vi "network_apply.vi"(8 "error":errorcluster, 11 "connection ID":refnum<k5>) -> (0 "error out":errorcluster, 3 "connection ID out":refnum<k5>)   [LabVIEW 2016, in "sen_api.lvlib"]
doc: "Applies the temporary IP configuration and loads it."
uses:
  sen_api.lvlib
panel:
  out "jsonRespIn":string
  out "JSON-response":string="{\"jsonrpc\":\"2.0\",\"method\":\"\",\"params\":[5,1.245,true,\"name\"],\"id\":\"1\"}"
  out "JSON request":string
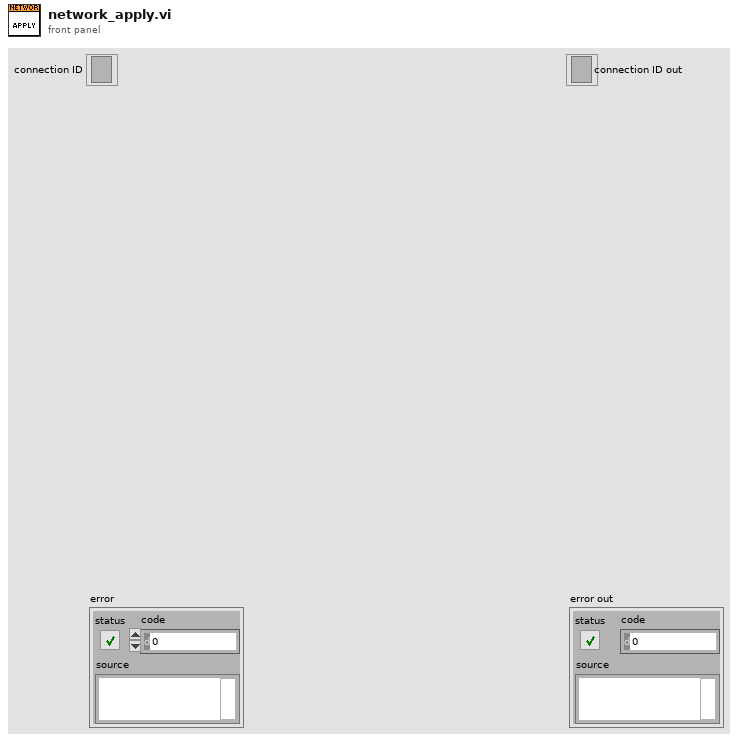
[diagram p1: front panel]
types:
  T1 = cluster{"jsonrpc":string, "method":string, "params":string[], "id":string, "api":i32, "pid":string}
  T2 = enum16{"Standard", "Buffered", "CRLF", "Immediate"}
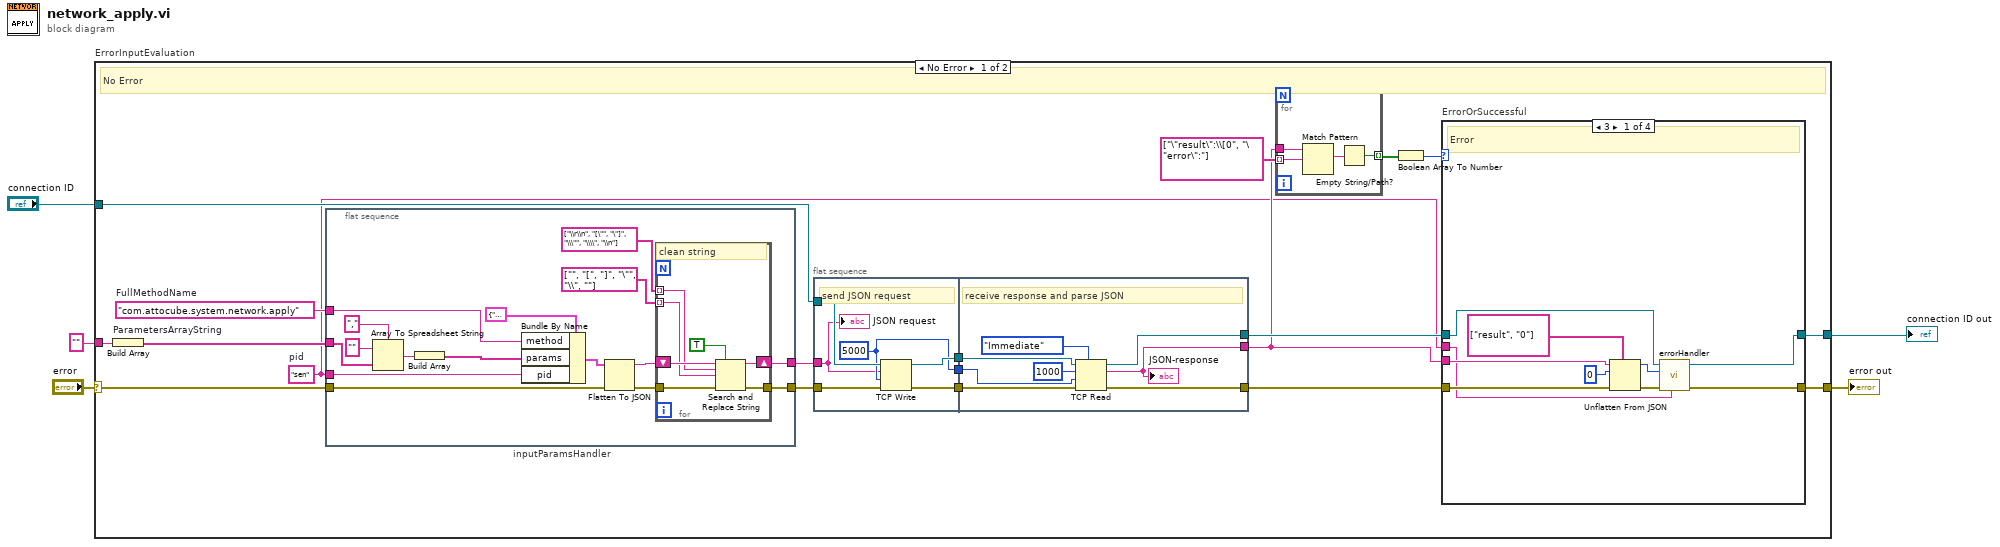
[diagram p0: block diagram]
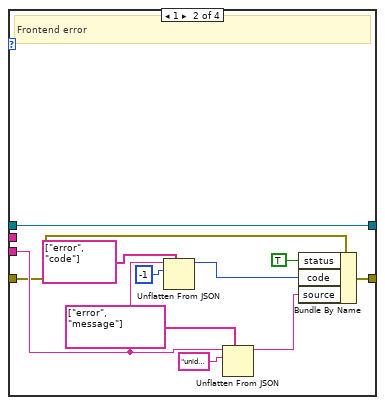
[diagram p2: hidden frame]
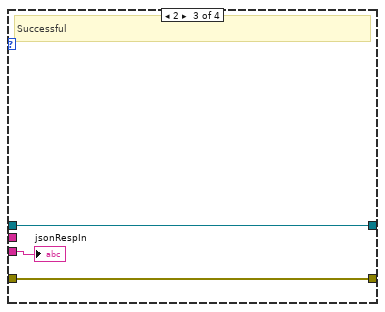
[diagram p3: hidden frame]
diagram:
  n1 = case "ErrorInputEvaluation" shown="No Error" "error" {
    selector: "error" -> [w11 w92]
    tunnel: "connection ID" -> [w21 w93]
    tunnel: [w13 w92] -> w4
    tunnel: [w14 w93] -> w3
    tunnel: "" -> [w6 _]
    frame No Error {
      w7 = "sen"  # pid
      w12 = "com.attocube.system.network.apply"  # FullMethodName
      # "No Error"
      n2 = Build Array "ParametersArrayString"(w6) -> (w10:string[])
      n3 = flat-sequence "inputParamsHandler" {
        tunnel: [w28] -> w9
        tunnel: w10 -> [w35]
        tunnel: w11 -> [w33]
        tunnel: [w30] -> w8
        tunnel: w12 -> [w36]
        tunnel: w7 -> [w25]
        frame #0 {
          n4 = Array To Spreadsheet String(delimiter (Tab)=",", array=w35, 3:"" ("format string")) -> (spreadsheet string=w38:string)
          n5 = Build Array "Build Array"(w38) -> (w34:string[])
          n6 = Bundle By Name(cluster=T1 {"jsonrpc"="2.0", "method"="com.attocube.amc.res.setRESReadOutFreq", "params"=[], "id"="1", "api"=2, "pid"=""}, "method"=w36, "params"=w34, "pid"=w25) -> (w37:T1)
          n7 = Flatten To JSON(anything=w37, error in (no error)=w33) -> (JSON string=w29:string, 11:w31:errorcluster)  [unwired: 1 in]
          n8 = for {
            tunnel: string[] ["\\r\\n", "[\"", "\"]", "\\\"", "\\\\", "\\n"] ("search string") -> [w44] mode=indexing
            tunnel: string[] ["", "[", "]", "\"", "\\", ""] ("replace string (\"\")") -> [w43] mode=indexing
            shift-right: [w46] -> w28
            shift-left: w29 -> [w45]
            tunnel: w31 -> [w42]
            tunnel: [w41] -> w30
            # "clean string"
            n9 = Search and Replace String(replace all?=TRUE ("replace all? (F)"), input string=w45, search string=w44, replace string=w43, error in=w42) -> (result string=w46:string, error out=w41:errorcluster)  [unwired: 3 in, 2 out]
          }
        }
      }
      n10 = flat-sequence {
        tunnel: w21 -> [w83]
        tunnel: [w81] -> w24
        tunnel: [w82] -> w23
        tunnel: w8 -> [w78]
        tunnel: [w80] -> w22
        tunnel: w9 -> [w79]
        tunnel: [w87] -> w17
        tunnel: w24 -> [w89]
        tunnel: w23 -> [w88]
        tunnel: [w85] -> w16
        tunnel: w22 -> [w86]
        tunnel: [w84] -> w15
        frame #0 {
          w80 = 5000 ("timeout ms (25000)")
          # "send JSON request"
          n11 = TCP Write(connection ID=w83, data in=w79, error in (no error)=w78, 9:w80) -> (connection ID out=w81:refnum<k5>, error out=w82:errorcluster)  [unwired: 1 out]
          "JSON request" <- w79
        }
        frame #1 {
          # "receive response and parse JSON"
          n12 = TCP Read(connection ID=w89, bytes to read=1000, error in (no error)=w88, 7:T2."Immediate" ("mode (standard)"), 9:w86) -> (connection ID out=w87:refnum<k5>, data out=w84:string, error out=w85:errorcluster)
          "JSON-response" <- w84
        }
      }
      n13 = for {
        tunnel: string[] ["\"result\":\\[0", "\"error\":"] ("path") -> [w50] mode=indexing
        tunnel: [w48] -> w19 mode=indexing
        tunnel: w15 -> [w51]
        n14 = Match Pattern(string=w51, regular expression=w50) -> (match substring=w49:string)  [unwired: 1 in, 3 out]
        n15 = Empty String/Path?(string/path=w49) -> (empty?=w48:bool)
      }
      n16 = Boolean Array To Number(Boolean array=w19) -> (number=w18:u32)
      n17 = case "ErrorOrSuccessful" shown="3" w18 {
        tunnel: w15 -> [w55 w64 w73 _]
        tunnel: w17 -> [w59 w62 w75 w77]
        tunnel: [w57 w62 w75 w77] -> w14
        tunnel: [w58 w65 w74 w76] -> w13
        tunnel: w16 -> [w61 w63 w74 w76]
        tunnel: w7 -> [w52 _ _ _]
        frame 3 {
          # "Error"
          n18 = Unflatten From JSON(path=string[] ["result", "0"], JSON string=w55, type and defaults=0, error in (no error)=w61) -> (value=w53:i32, error out=w60:errorcluster)  [unwired: 3 in]
          n19 = call "errorHandler.vi"("pid"=w52, "error in"=w60, "errNbr"=w53, "connection ID"=w59) -> ("error out 2"=w58:errorcluster, "connection ID out"=w57:refnum<k5>)  [unwired: 6 in]
        }
        frame 1 {
          # "Frontend error"
          n20 = Unflatten From JSON(path=string[] ["error", "code"], JSON string=w64, type and defaults=-1) -> (value=w71:i32)  [unwired: 4 in, 1 out]
          n21 = Unflatten From JSON(path=string[] ["error", "message"], JSON string=w64, type and defaults="unidentified error") -> (value=w72:string)  [unwired: 4 in, 1 out]
          n22 = Bundle By Name(cluster=w63, "status"=TRUE, "code"=w71, "source"=w72) -> (w65:errorcluster)
        }
        frame 2 {
          # "Successful"
          "jsonRespIn" <- w73
        }
        frame Default {
          # "NoResponse"
        }
      }
    }
    frame Error {
      # "Error"
    }
  }
  "error out" <- w4
  "connection ID out" <- w3
